vi "GetMeasureExecutionStatus.vi"(8 "error in":errorcluster, 11 "Measure in":refnum<class "Measure.lvclass">) -> (0 "error out":errorcluster, 2 "MeasureExecutionStatus":T1, 3 "Measure out":refnum<class "Measure.lvclass">)   [LabVIEW 2021, in "ProligentXMLGenerator.lvlib" / "Measure.lvclass"]
doc: "Define the execution status of the measure\n\nPASS: The execution completed successfully.\nFAIL: The execution completed and failures were detected.\nNOT_COMPLETED: The execution is not completed. It is still in progress. In that situation, the end time of the execution must be ommited.\nABORTED: The execution was aborted."
uses:
  Measure.lvclass
  Measure.lvclass/Measure.ctl
  Base/ExecutionStatus/ExecutionStatus.lvclass
  Base/ExecutionStatus/Value.ctl
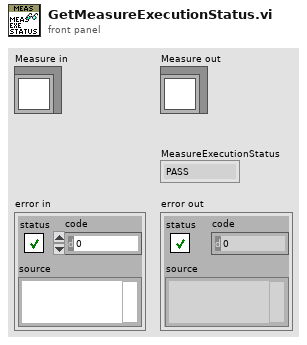
[diagram p1: front panel]
types:
  T1 = typedef "ProligentXMLGenerator.lvlib/ExecutionStatus.lvclass/Value.ctl" = enum16{"PASS", "FAIL", "NOT_COMPLETED", "ABORTED"}
  T2 = typedef "ProligentXMLGenerator.lvlib/Measure.lvclass/Data.ctl" = cluster{"Name":string, "Type":refnum<class "MeasureKind.lvclass">, "Precision":refnum<class "UnsignedByte.lvclass">, "Limit":refnum<class "MeasureLimit.lvclass">, "Characteristics":refnum<class "Characteristic.lvclass">[], "FailureReferences":refnum<class "FailureReference.lvclass">[], "CustomData":refnum<class "CustomData.lvclass">, "MeasureId":refnum<class "Guid.lvclass">, "MeasureTime":refnum<class "DateTime.lvclass">, "Comments":refnum<class "NonNullableString_TruncateAt_255.lvclass">, "Unit":refnum<class "NonEmptyString_30.lvclass">, "Symbol":refnum<class "NonEmptyString_20.lvclass">, "MeasureExecutionStatus":refnum<class "ExecutionStatus.lvclass">}
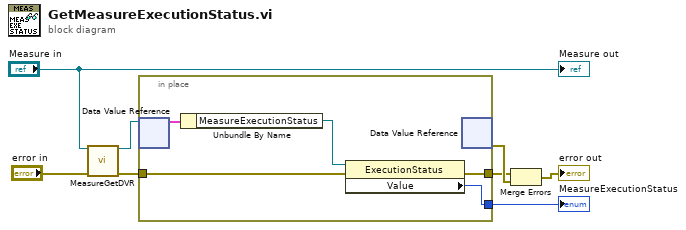
[diagram p0: block diagram]
diagram:
  n1 = call "MeasureGetDVR.vi"("error in"="error in", "Measure"="Measure in") -> ("error out"=w2:errorcluster, "DVRReference"=w7:refnum<data-value>)  [unwired: 8 in]
  n2 = in-place "In Place Element Structure" {
    in-place-border: [w10] -> w6
    in-place-border: w2 -> [w11]
    in-place-border: [w9] -> w1
    n3 = in-place-dvr #1(w7) -> (w13:T2)  [unwired: 1 out]
    n4 = Unbundle By Name(w13) -> ("MeasureExecutionStatus"=w12:refnum<class "ExecutionStatus.lvclass">)
    n5 = property on="Property Node" class="ExecutionStatus"(reference=w12, error in=w11) -> (error out=w9:errorcluster, "Value"=w10:T1)  [unwired: 1 out]
    n6 = in-place-dvr #1() -> (w8:errorcluster)  [unwired: 1 in, 1 out]
  }
  "MeasureExecutionStatus" <- w6
  n7 = Merge Errors(w1, w8) -> (→"error out":errorcluster)
  "Measure out" <- "Measure in"
